vi "GetAxisValuesII (SubVI).vi"(11 "read buffer":string) -> (3 "Array":dbl[](array[numeric]))   [LabVIEW 2024]
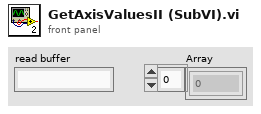
[diagram p1: front panel]
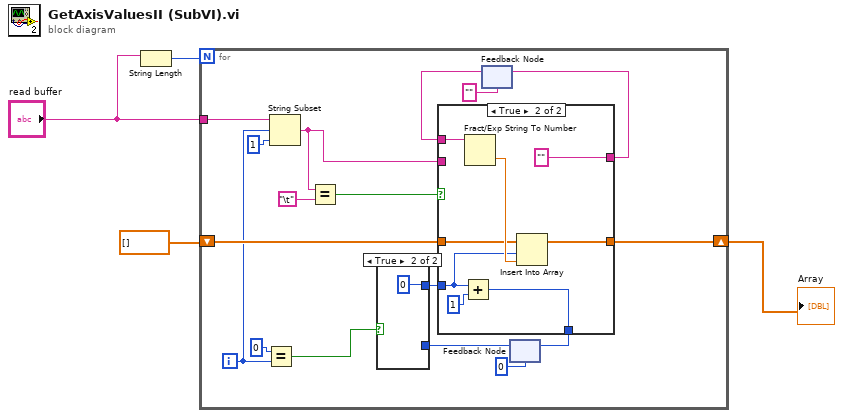
[diagram p0: block diagram]
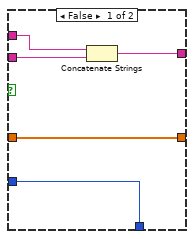
[diagram p3: hidden frame]
diagram:
  n1 = String Length(string="read buffer") -> (length=w2:i32)
  n2 = for {
    N: w2 -> [_]
    tunnel: "read buffer" -> [w20]
    shift-right: [w15] -> w4
    shift-left: dbl[] [] -> [w12]
    i -> [w11]
    n3 = Equal?(x=0, y=w11) -> (x = y?=w9:bool)
    n4 = String Subset(string=w20, offset (0)=w11, length (rest)=1 ("Länge (Rest)")) -> (substring=w13:string)
    n5 = Equal?(x=w13, y="\t") -> (x = y?=w6:bool)
    n6 = feedback #1("") -> (w17:string)
    n7 = feedback #2(0) -> (w8:i32)
    n8 = case shown="True" w9 {
      tunnel: w8 -> [w22 _]
      tunnel: [w22 0] -> w7
      frame False {
      }
      frame True {
      }
    }
    n9 = case shown="True" w6 {
      tunnel: w7 -> [w24 w31]
      tunnel: w13 -> [w27 _]
      tunnel: w17 -> [w28 w34]
      tunnel: [w26 ""] -> w18
      tunnel: w12 -> [w25 w30]
      tunnel: [w25 w33] -> w15
      tunnel: [w24 w29] -> w5
      frame False {
        n10 = Concatenate Strings(w28, w27) -> (w26:string)
      }
      frame True {
        n11 = Add(x=w31, y=1) -> (x+y=w29:i32)
        n12 = Fract/Exp String To Number(string=w34) -> (number=w32:dbl)  [unwired: 3 in, 1 out]
        n13 = Insert Into Array(array=w30, index=w31, new element=w32) -> (w33:dbl[])
      }
    }
    n14 = feedback-in #1(w18) -> ()
    n15 = feedback-in #2(w5) -> ()
  }
  "Array" <- w4
